vi "Attacker.vi"(0 "command\nenum":T7, 1 "IA State Input 2":T3={"our_robots"=[], "enemy_robots"=[], "balls"=[], "geometry"={"line_width"=0, "field_length"=0, "field_width"=0, "boundary_width"=0, "referee_width"=0, "goal_width"=0, "goal_depth"=0, "goal_wall_width"=0, "center_circle_radius"=0, "defense_radius"=0, "defense_stretch"=0, "free_kick_from_defense_dist"=0, "penalty_spot_from_field_line_dist"=0, "penalty_line_from_spot_dist"=0}, "IA Judge"={"stage"="", "command"="", "our_goalie_id"=0.0, "enemy_goalie_id"=0.0, "command\nenum"=enum."Halt", "Time"=enum."Azul"}, "Received Timestamp"=timestamp(0 s since 1904-01-01), "Events"={"Touch"=FALSE, "Ball out"=FALSE, "id touch"=0.0, "Ball out of \nVision"=FALSE, "Ball inside \nGoalie area"=FALSE, "Robot not responding"=FALSE, "Robots responding status"=[1.0, 1.0, 1.0, 1.0, 1.0, 1.0]}}, 2 "Total de robos":u32[](array[numeric]), 5 "Robot in":T1, 7 "Opponent goalie":T1, 11 "atacando contra?":bool=TRUE, 12 "geometry":T5, 14 "balls":T4[](array[typedef])) -> (6 "output cluster":T1)   [LabVIEW 2016]
uses:
  Command Enum.ctl
  Core/AI Robot.ctl
  Functions Enum.ctl
  Core/Field Size.ctl
  Core/AI Ball.ctl
  Core/AI Input.ctl
  Core/AI Judge.ctl
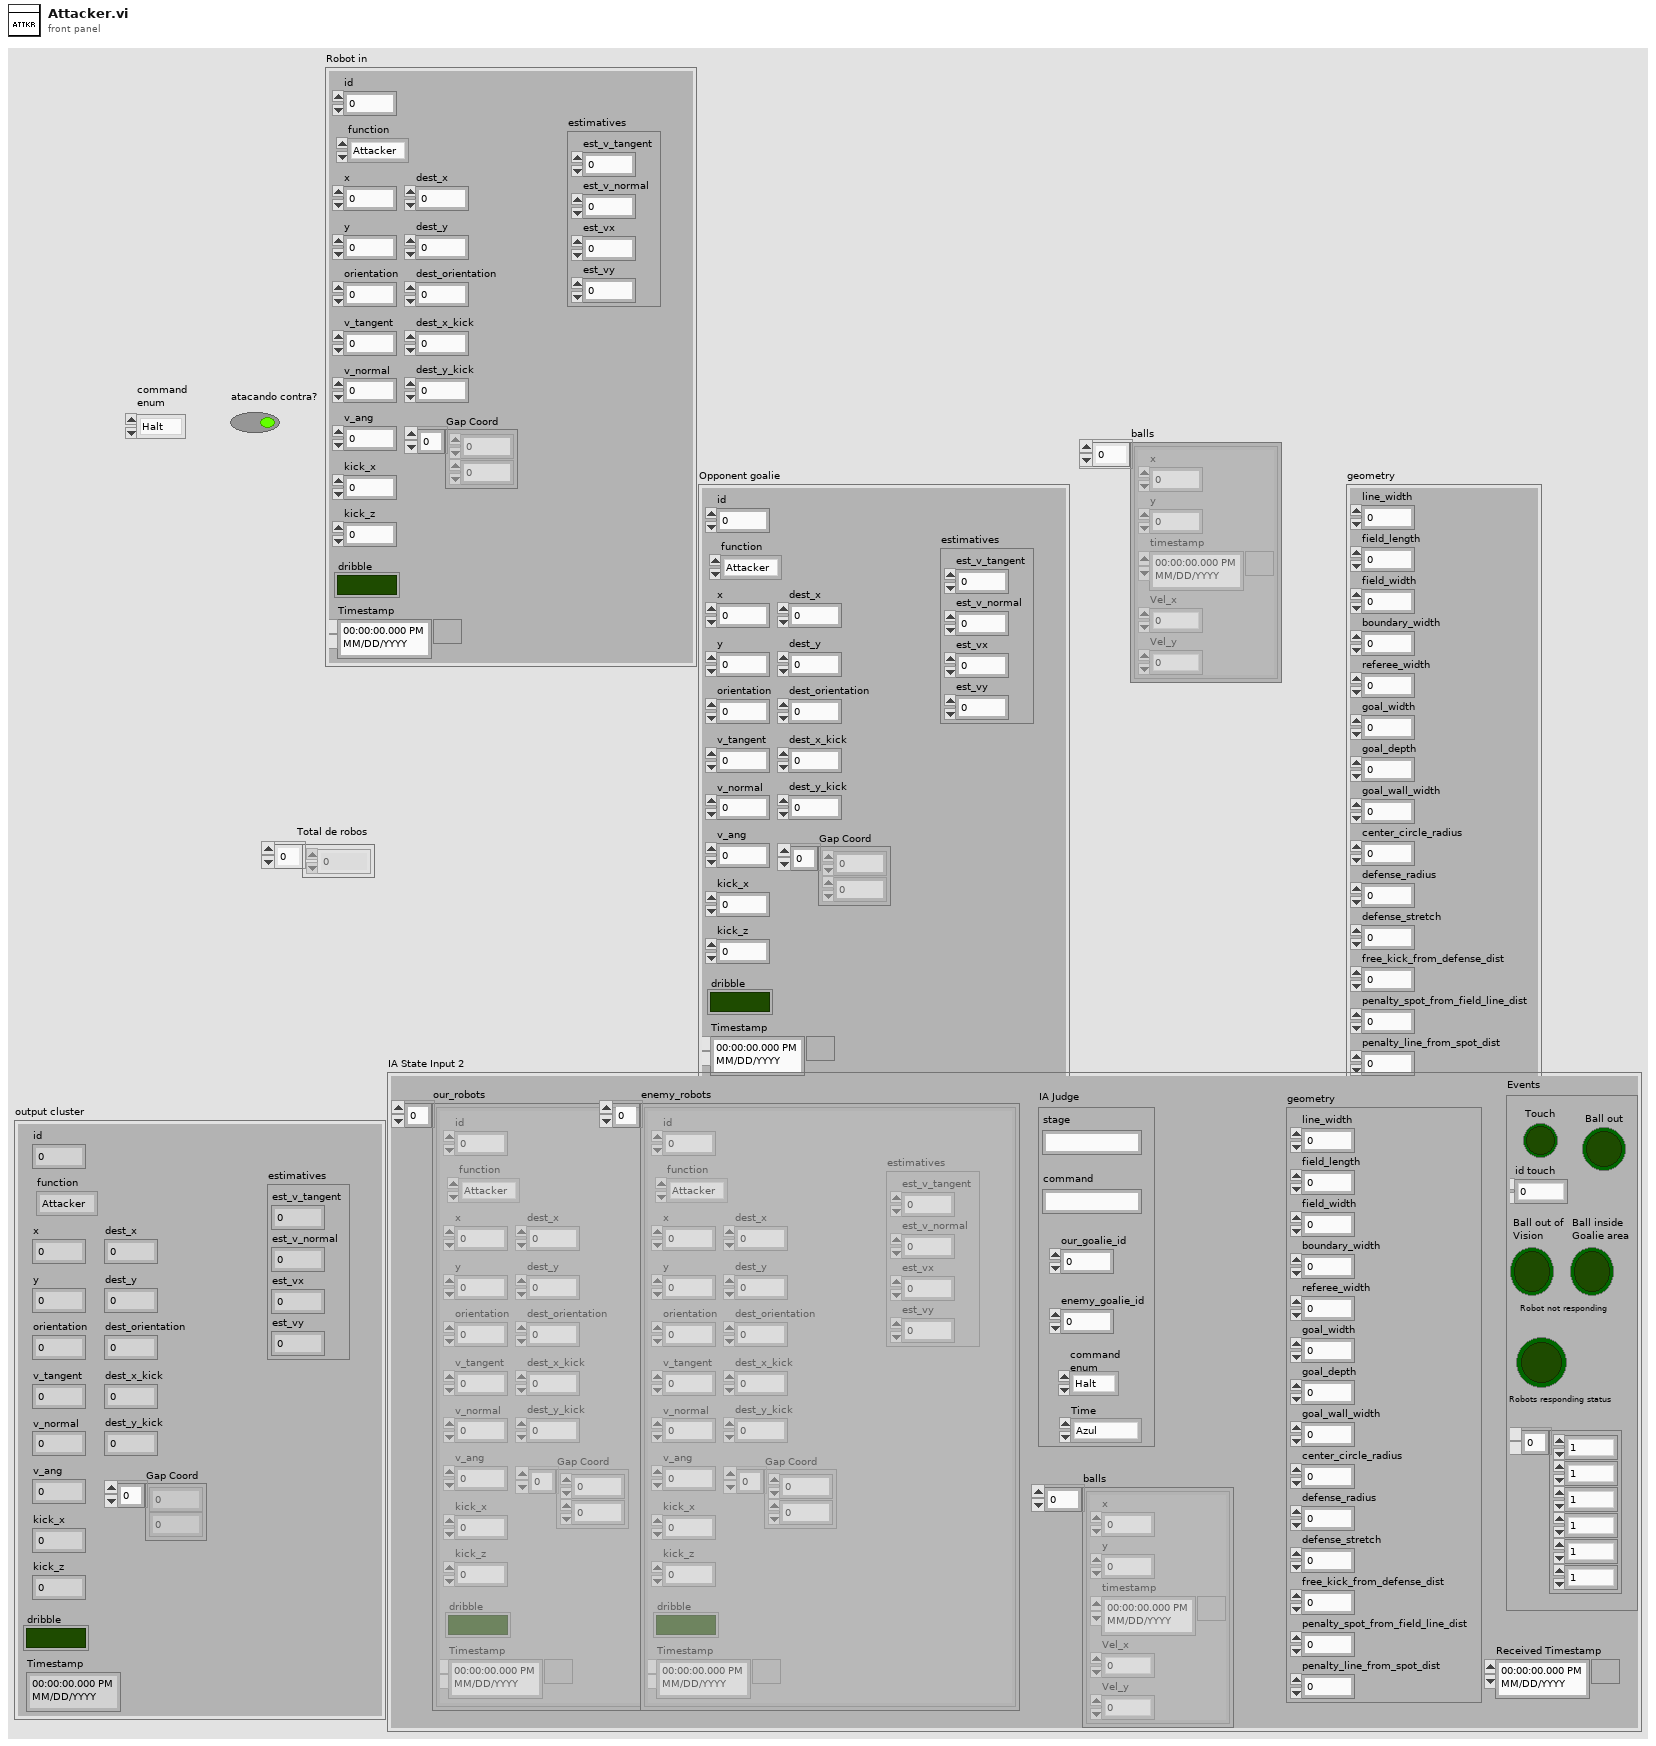
[diagram p1: front panel]
types:
  T1 = typedef "AI Robot.ctl" = cluster{"id":u32, "function":T2, "x":dbl, "y":dbl, "orientation":dbl, "v_tangent":dbl, "v_normal":dbl, "v_ang":dbl, "kick_x":dbl, "kick_z":dbl, "dribble":bool, "Timestamp":timestamp, "dest_x":dbl, "dest_y":dbl, "dest_orientation":dbl, "estimatives":cluster{"est_v_tangent":dbl, "est_v_normal":dbl, "est_vx":dbl, "est_vy":dbl}, "dest_x_kick":dbl, "dest_y_kick":dbl, "Gap Coord":dbl[]}
  T2 = typedef "Functions Enum.ctl" = enum16{"Attacker", "Goalie", "Defender", "Striker", "Goto 0", "Dummy", "Kicker", "ZigZag"}
  T3 = typedef "AI Input.ctl" = cluster{"our_robots":T1[], "enemy_robots":T1[], "balls":T4[], "geometry":T5, "IA Judge":T6, "Received Timestamp":timestamp, "Events":cluster{"Touch":bool, "Ball out":bool, "id touch":dbl, "Ball out of \nVision":bool, "Ball inside \nGoalie area":bool, "Robot not responding":bool, "Robots responding status":dbl[]}}
  T4 = typedef "AI Ball.ctl" = cluster{"x":dbl, "y":dbl, "timestamp":timestamp, "Vel_x":dbl, "Vel_y":dbl}
  T5 = typedef "Field Size.ctl" = cluster{"line_width":u32, "field_length":u32, "field_width":u32, "boundary_width":u32, "referee_width":u32, "goal_width":u32, "goal_depth":u32, "goal_wall_width":u32, "center_circle_radius":u32, "defense_radius":u32, "defense_stretch":u32, "free_kick_from_defense_dist":u32, "penalty_spot_from_field_line_dist":u32, "penalty_line_from_spot_dist":u32}
  T6 = typedef "AI Judge.ctl" = cluster{"stage":string, "command":string, "our_goalie_id":dbl, "enemy_goalie_id":dbl, "command\nenum":T7, "Time":enum16{"Azul", "Amarelo"}}
  T7 = typedef "Command Enum.ctl" = enum16{"Halt", "Stop", "Force Start", "PKA Normal Start", "Prepare Kickoff Ally", "PKE Normal Start", "Prepare Kickoff Enemy", "Prepare Penalty Ally", "PPA Normal Start", "Prepare Penalty Enemy", "PPE Normal Start", "Direct Free Enemy", "Direct Free Ally", "Indirect Free Enemy", "Indirect Free Ally", "Timeout Enemy", "Timeout Ally", "Goal Enemy", "Goal Ally", "Ball Placement Enemy", "Ball Placement Ally", "None"}
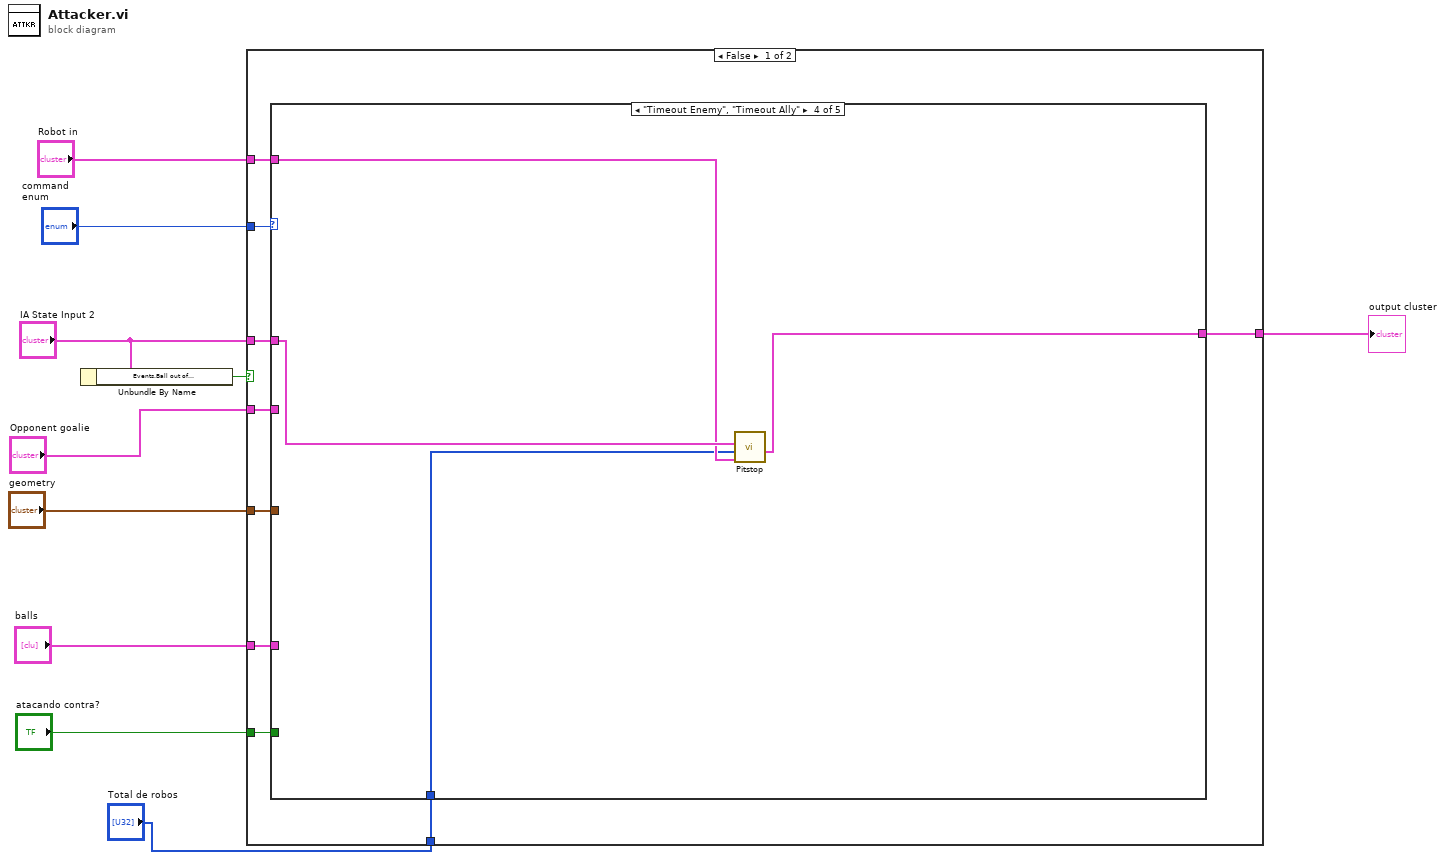
[diagram p0: block diagram]
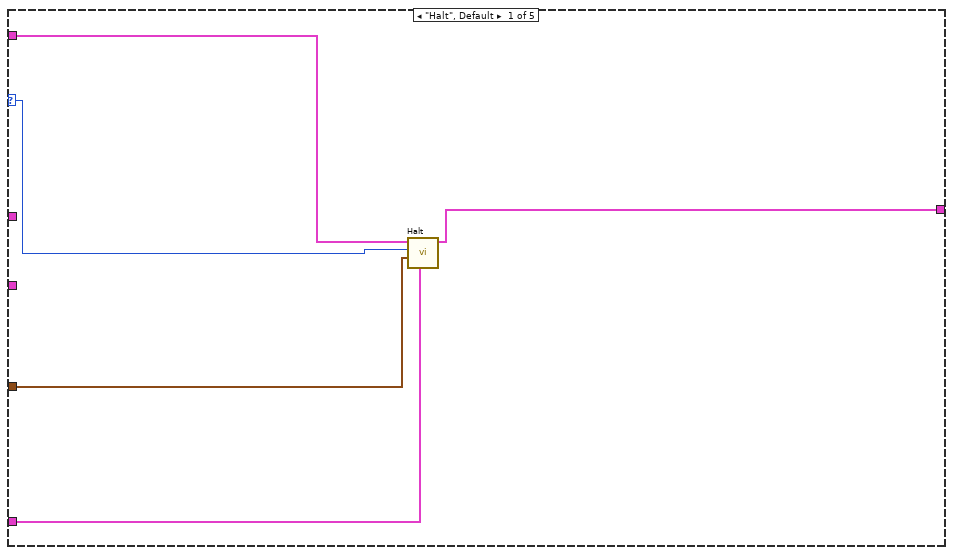
[diagram p2: hidden frame]
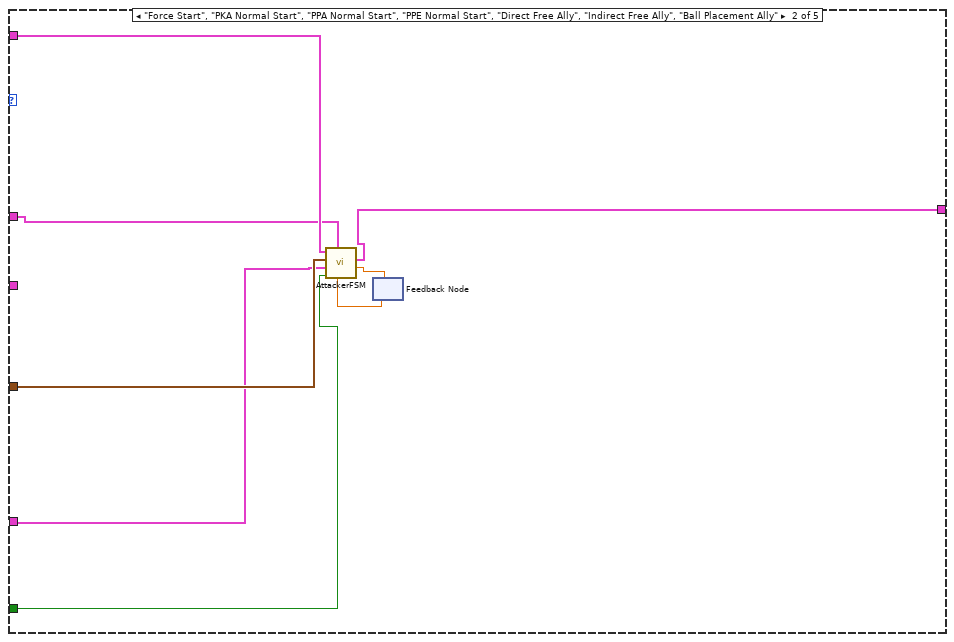
[diagram p3: hidden frame]
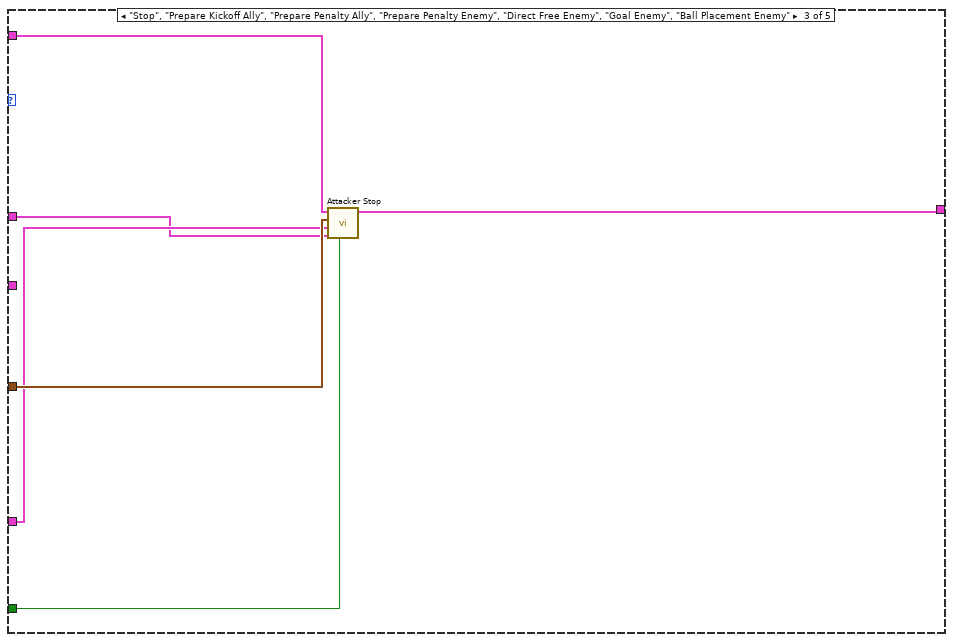
[diagram p4: hidden frame]
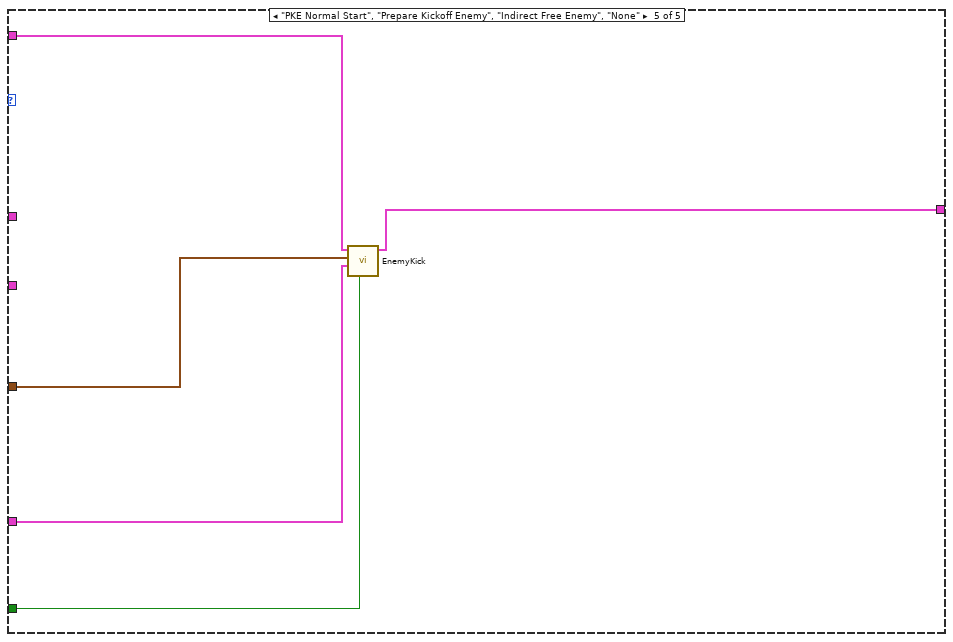
[diagram p5: hidden frame]
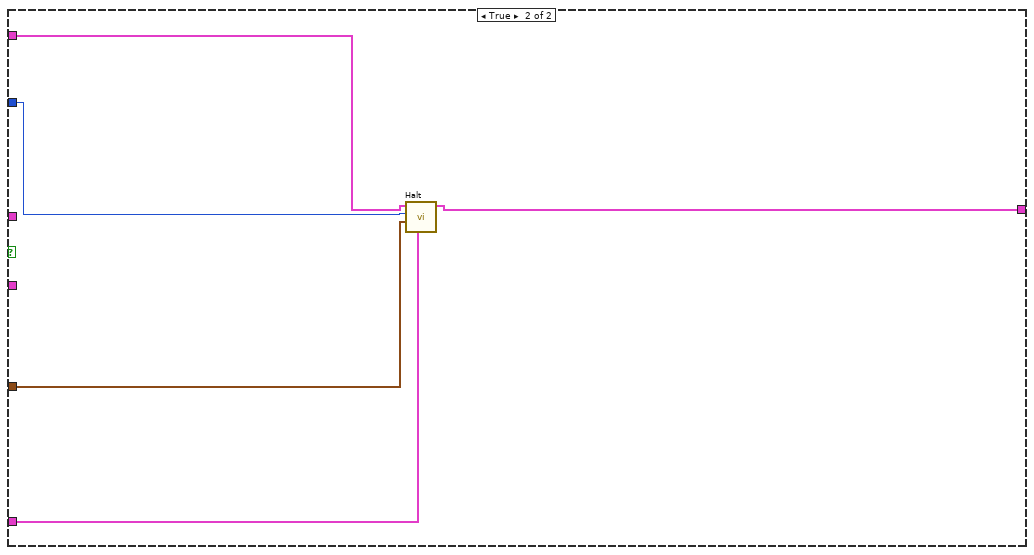
[diagram p6: hidden frame]
diagram:
  n1 = Unbundle By Name("IA State Input 2") -> ("Events.Ball out of \nVision"=w2:bool)
  n2 = case shown="False" w2 {
    tunnel: "command\nenum" -> [w19 w50]
    tunnel: [w18 w52] -> w9
    tunnel: "Opponent goalie" -> [w17 _]
    tunnel: "geometry" -> [w16 w49]
    tunnel: "balls" -> [w15 w48]
    tunnel: "atacando contra?" -> [w14 _]
    tunnel: "Robot in" -> [w13 w51]
    tunnel: "IA State Input 2" -> [w12 _]
    tunnel: "Total de robos" -> [w11 _]
    frame False {
      n3 = case shown="\"Timeout Enemy\", \"Timeout Ally\"" w19 {
        selector: w19 -> [w22 _ _ _ _]
        tunnel: [w24 w30 w36 w40 w47] -> w18
        tunnel: w17 -> [_ _ _ _ _]
        tunnel: w16 -> [w21 w32 w38 _ w44]
        tunnel: w15 -> [w20 w31 w37 _ w46]
        tunnel: w14 -> [_ w27 w33 _ w45]
        tunnel: w13 -> [w23 w26 w35 w41 w43]
        tunnel: w12 -> [_ w25 w34 w42 _]
        tunnel: w11 -> [_ _ _ w39 _]
        frame "Halt", Default {
          n4 = call "Halt.vi"("balls"=w20, "Field Size in"=w21, "Numeric"=w22, "Robot in"=w23) -> ("Robot out"=w24:T1)  [unwired: 7 in]
        }
        frame "Force Start", "PKA Normal Start", "PPA Normal Start", "PPE Normal Start", "Direct Free Ally", "Indirect Free Ally", "Ball Placement Ally" {
          n5 = feedback #1() -> (w28:dbl)  [unwired: 1 in]
          n6 = call "AttackerFSM.vi"("Current State"=w28, "IA State Input 2"=w25, "atacando contra?"=w27, "balls"=w31, "Field Size in"=w32, "Robot in"=w26) -> ("Next State"=w29:dbl, "Robot out"=w30:T1)  [unwired: 4 in]
          n7 = feedback-in #1(w29) -> ()
        }
        frame "Stop", "Prepare Kickoff Ally", "Prepare Penalty Ally", "Prepare Penalty Enemy", "Direct Free Enemy", "Goal Enemy", "Ball Placement Enemy" {
          n8 = call "Attacker Stop.vi"("atacando contra?"=w33, "IA State Input 2"=w34, "balls"=w37, "Field Size in"=w38, "Robot in"=w35) -> ("Robot out"=w36:T1)  [unwired: 6 in]
        }
        frame "Timeout Enemy", "Timeout Ally" {
          n9 = call "Pitstop.vi"("Robot in"=w41, "robos"=w39, "IA State Input"=w42) -> ("Robot out"=w40:T1)  [unwired: 8 in]
        }
        frame "PKE Normal Start", "Prepare Kickoff Enemy", "Indirect Free Enemy", "None" {
          n10 = call "EnemyKick.vi"("atacando contra?"=w45, "balls"=w46, "Field Size in"=w44, "Robot in"=w43) -> ("Robot out"=w47:T1)  [unwired: 7 in]
        }
      }
    }
    frame True {
      n11 = call "Halt.vi"("balls"=w48, "Field Size in"=w49, "Numeric"=w50, "Robot in"=w51) -> ("Robot out"=w52:T1)  [unwired: 7 in]
    }
  }
  "output cluster" <- w9
